vi "GV-Selprops-global.vi"() -> ()   [LabVIEW 2020, in "Sgraph_lib_V1.lvlib"]
uses:
  Builds/Sgraph_lib_V1.lvlib
  Gview/controls/Typedef_SelProperties.ctl
  Gview/controls/Typedef_LineType.ctl
  Gview/Gviewer.lvclass
panel:
  in  "OS":dbl
  in  "Gain":dbl
  in  "Bottom":dbl
  in  "TOP":dbl
  out "SelProperties":T1[](array[typedef])
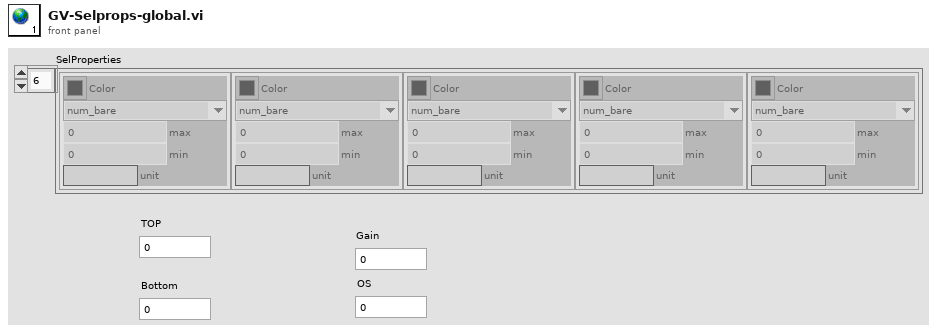
[diagram p1: front panel]
types:
  T1 = typedef "Sgraph_lib_V1.lvlib/Gviewer.lvclass/Typedef_SelProperties.ctl" = cluster{"Color":u32, "LineType":T2, "max":dbl, "min":dbl, "unit":string}
  T2 = typedef "Sgraph_lib_V1.lvlib/Gviewer.lvclass/Typedef_LineType.ctl" = enum16{"num_bare", "num_MinMax_Area", "num_MinMax_Lines", "num_MinMax_Forfor", "num_Max_Area", "num_Max_Line", "num_Max_Forfor", "num_Min_Area", "num_Min_Line", "num_Min_Fosfor", "Boolean_Line_01", "Boolean_Area_01", "Boolean_Fosfor_01", "Boolean_Line_TF", "Boolean_Area_TF", "Boolean_Fosfor_TF", "Boolean_OnOff_Line", "Boolean_OnOff_Area", "Boolean_OnOff_Fosfor", "Boolean_spare", "StringEvent_Line", "StringEvent_TimeLine"}
diagram:
